vi "DrawDotsXY.vi"(6 "color":u32(colorbox)=51250, 7 "Empty picture":picture, 8 "fill?(F)":bool, 9 "radius":i16=2, 10 "new position":cluster{"x":i16, "y":i16}, 11 "Array":dbl[][](array[numeric])) -> (3 "2D picture":picture)   [LabVIEW 2024]
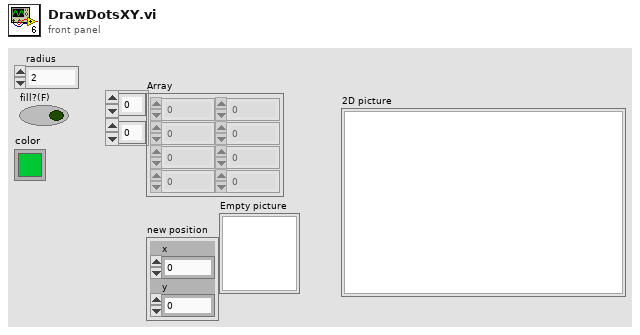
[diagram p1: front panel]
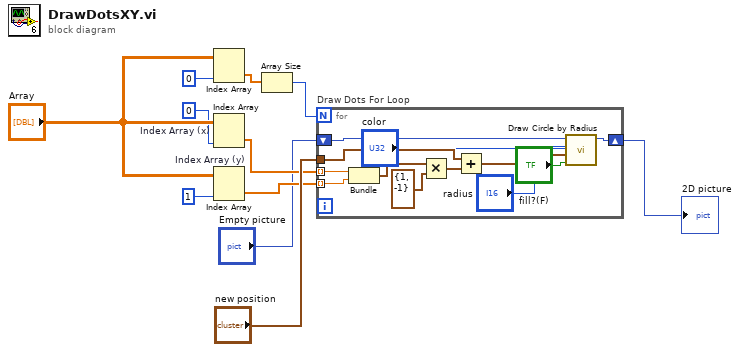
[diagram p0: block diagram]
diagram:
  n1 = Index Array "Index Array"(array="Array", index (col)=0 ("index (row)")) -> (element=w2:dbl[])  [unwired: 1 in]
  n2 = Index Array "Index Array (x)"(array="Array", index (col)=0 ("index (row)")) -> (element=w4:dbl[])  [unwired: 1 in]
  n3 = Index Array "Index Array (y)"(array="Array", index (col)=1 ("index (row)")) -> (element=w5:dbl[])  [unwired: 1 in]
  n4 = Array Size(array=w2) -> (size(s)=w3:i32)
  n5 = for "Draw Dots For Loop" {
    N: w3 -> [_]
    tunnel: w4 -> [w21] mode=indexing
    tunnel: w5 -> [w20] mode=indexing
    shift-right: [w19] -> w9
    shift-left: "Empty picture" -> [w18]
    tunnel: "new position" -> [w14]
    n6 = Bundle("x2"=w21, "x2"=w20) -> (w16:cluster{"x2":dbl, "x2":dbl})  [unwired: 1 in]
    n7 = Multiply(x=w16, y=cluster{"x":i16, "y":i16} {"x"=1, "y"=-1} ("new position")) -> (x*y=w15:cluster{dbl, dbl})
    n8 = Add(x=w14, y=w15) -> (x+y=w13:cluster{dbl, dbl})
    n9 = call <vilib>:"Draw Circle by Radius.vi"("color(black)"="color", "fill?(F)"="fill?(F)", "pixel center"=w13, "radius"="radius", "picture"=w18) -> ("new picture"=w19:picture)  [unwired: 6 in]
  }
  "2D picture" <- w9
